vi "Lookup Array Element (Hierarchy).vi"(8 "error in (no error)":errorcluster, 9 "Index":i32, 10 "Hierarchy":string[](array[string]), 11 "TemplateLocals in":refnum<class "Value Tree.lvclass">) -> (0 "error out":errorcluster, 1 "Value":string, 2 "Type":T1, 3 "TemplateLocals out":refnum<class "Value Tree.lvclass">, 4 "Children":string[](array[string]), 5 "Size":i32)   [LabVIEW 2020, in "HTTP Server.lvlib" / "Value Tree.lvclass"]
uses:
  Value Tree.lvclass
  Value Tree.lvclass/Value Tree.ctl
  Local Type.ctl
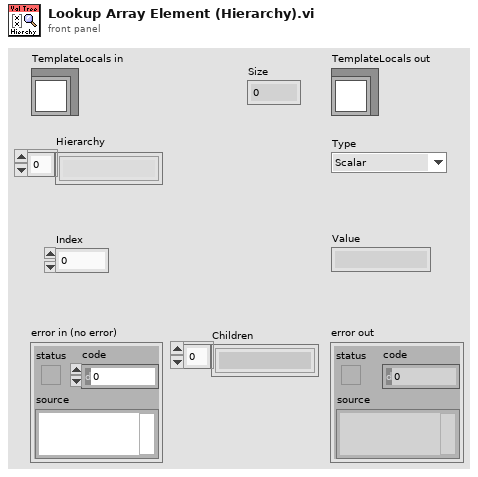
[diagram p1: front panel]
types:
  T1 = typedef "HTTP Server.lvlib/Value Tree.lvclass/Local Type.ctl" = enum16{"Scalar", "Object", "Array"}
  T2 = typedef "HTTP Server.lvlib/Value Tree.lvclass/Local Info.ctl" = cluster{"Type":T1, "Value":string, "Children":string[], "Size":i32}
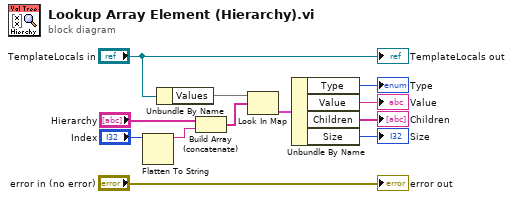
[diagram p0: block diagram]
diagram:
  n1 = Flatten To String(anything="Index") -> (data string=w8:string)  [unwired: 3 in, 2 out]
  n2 = Unbundle By Name("TemplateLocals in") -> ("Values"=w7:map{string[], T2})
  n3 = Build Array (concatenate)("Hierarchy", w8) -> (w6:string[])
  n4 = Look In Map(map=w7, key=w6) -> (value=w5:T2)  [unwired: 1 in, 1 out]
  n5 = Unbundle By Name(w5) -> ("Type"=→"Type":T1, "Value"=→"Value":string, "Children"=→"Children":string[], "Size"=→"Size":i32)
  "error out" <- "error in (no error)"
  "TemplateLocals out" <- "TemplateLocals in"
